vi "test - Empty String Check.vi"(8 "error in (no error)":errorcluster, 11 "TestCase in":refnum<class "testcase-Supported-Datatype.lvclass">) -> (0 "error out":errorcluster, 3 "TestCase out":refnum<class "testcase-Supported-Datatype.lvclass">)   [LabVIEW 2017, in "testcase-Supported-Datatype.lvclass"]
uses:
  testcase-Supported-Datatype.lvclass
  <vilib>/addons/_JKI Toolkits/VI Tester/TestCase.llb/TestCase.lvclass
  addons/API-String-Arugments-Support/API String Arguments Support.lvlib
  C:/Program Files (x86)/National Instruments/LabVIEW 2017/vi.lib/addons/_JKI Toolkits/VI Tester/TestCase.llb/TestCase.lvclass
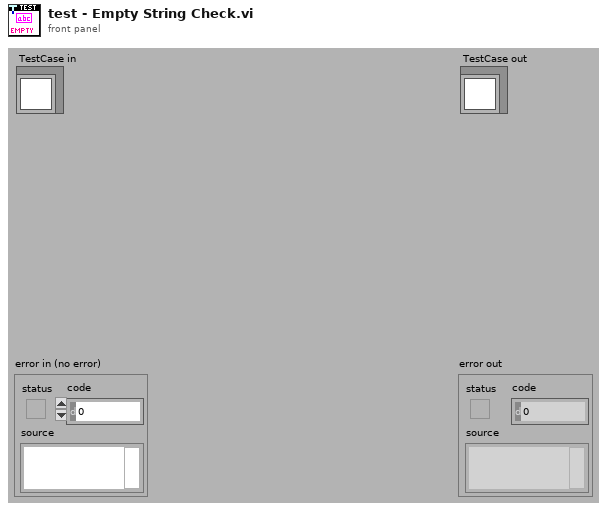
[diagram p1: front panel]
types:
  T1 = cluster{"Name":string, "Child":cluster{"Name":string}, "Bool":bool}[]
  T2 = cluster{"Name":string, "Child":cluster{"Name":string}, "Bool":bool}
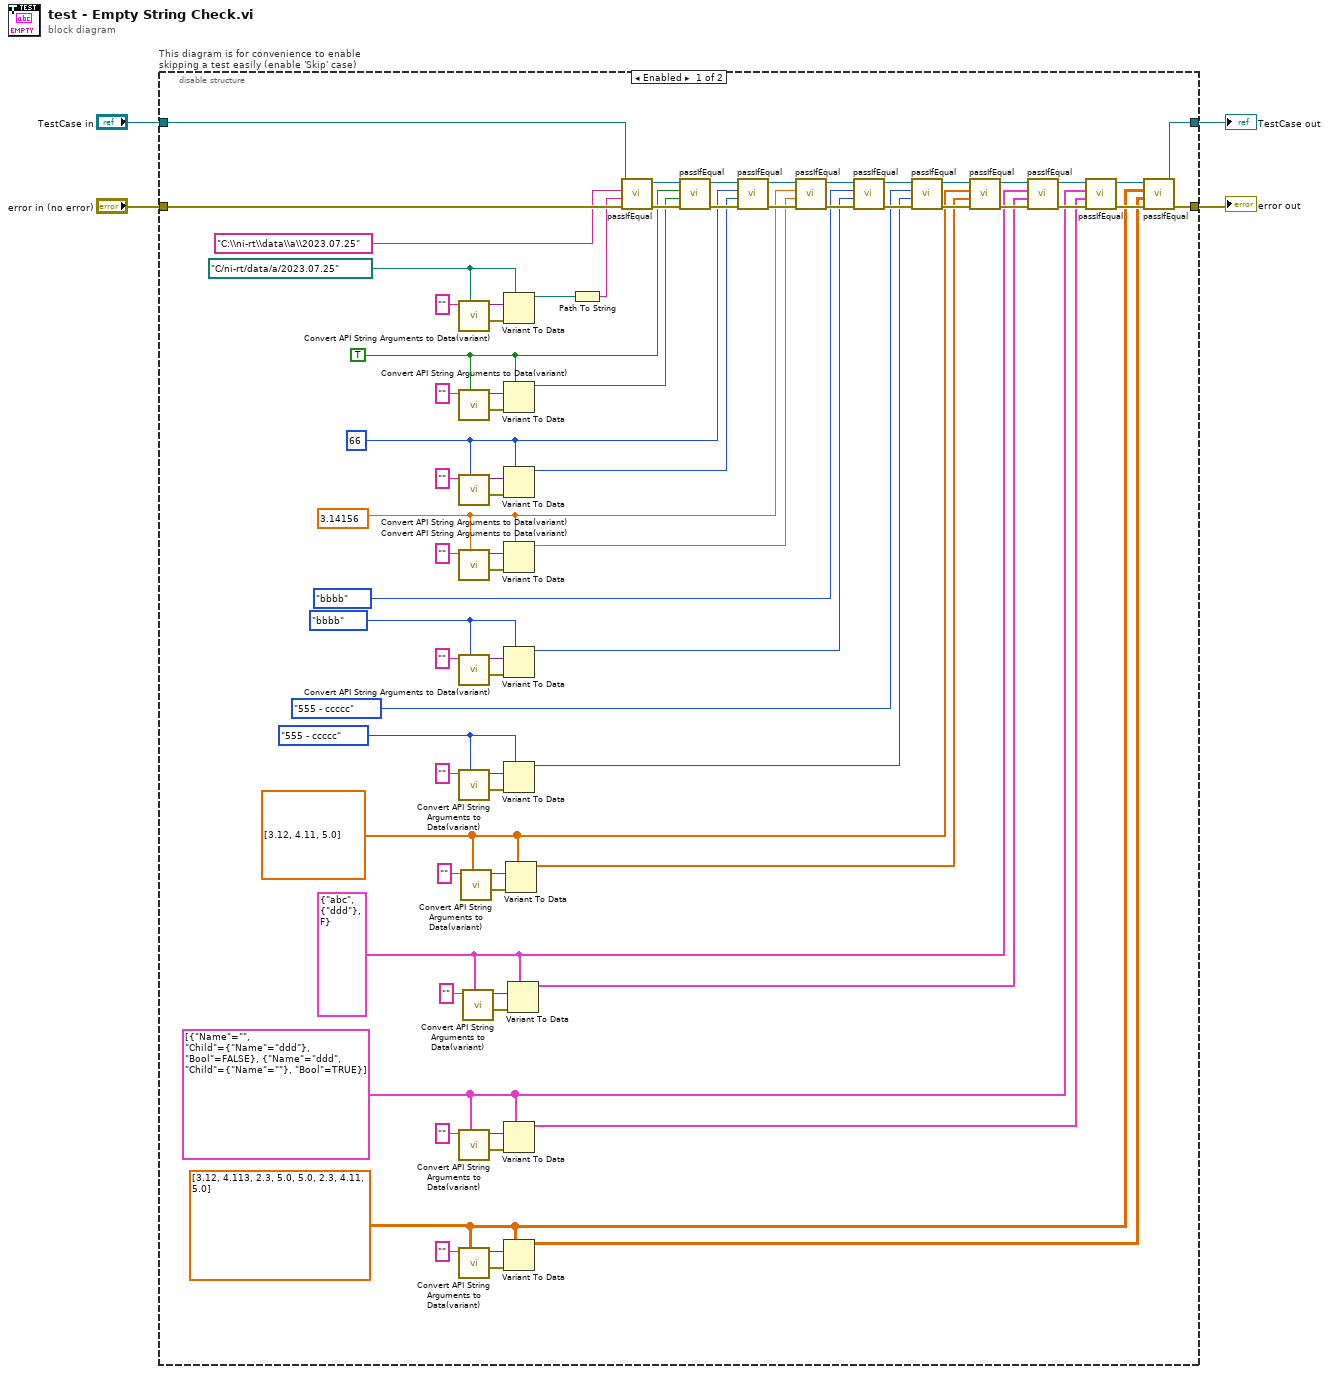
[diagram p0: block diagram]
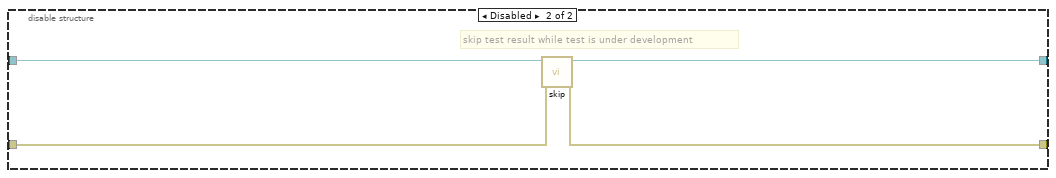
[diagram p2: hidden frame]
diagram:
  n1 = disable-structure "This diagram is for convenience to enable skipping a test easily (enable 'Skip' case)" shown="Enabled" {
    disable-tunnel: "TestCase in" -> [w80 w84]
    disable-tunnel: [w5 w82] -> w1
    disable-tunnel: [w6 w83] -> w3
    disable-tunnel: "error in (no error)" -> [w79 w81]
    frame Enabled {
      w8 = dbl[][] [[3.12, 4.113, 2.3, 5.0, 5.0, 2.3, 4.11, 5.0]] ("Data 11")
      w15 = T1 [{"Name"="", "Child"={"Name"="ddd"}, "Bool"=FALSE}, {"Name"="ddd", "Child"={"Name"=""}, "Bool"=TRUE}] ("Data 10")
      w22 = T2 {"Name"="abc", "Child"={"Name"="ddd"}, "Bool"=FALSE} ("Data 8")
      w29 = dbl[] [3.12, 4.11, 5.0] ("Data 4")
      w39 = enum16{"1 - aaaa", "2 - bbbb", "555 - ccccc"}."555 - ccccc" ("Data 6")
      w47 = enum16{"aaaa", "bbbb", "ccccc"}."bbbb" ("Data 5")
      w52 = 3.14156
      w59 = 66
      w66 = TRUE
      w75 = path "C:/ni-rt/data/a/2023.07.25" ("Data 9")
      n2 = call "Convert API String Arguments to Data(variant).vi"("Type"=w75, "String"="") -> ("error"=w78:errorcluster, "Data"=w77:variant)  [unwired: 8 in]
      n3 = call "Convert API String Arguments to Data(variant).vi"("Type"=w66, "String"="") -> ("error"=w71:errorcluster, "Data"=w70:variant)  [unwired: 8 in]
      n4 = call "Convert API String Arguments to Data(variant).vi"("Type"=w59, "String"="") -> ("error"=w62:errorcluster, "Data"=w63:variant)  [unwired: 8 in]
      n5 = call "Convert API String Arguments to Data(variant).vi"("Type"=w52, "String"="") -> ("error"=w57:errorcluster, "Data"=w56:variant)  [unwired: 8 in]
      n6 = call "Convert API String Arguments to Data(variant).vi"("Type"=w47, "String"="") -> ("error"=w50:errorcluster, "Data"=w49:variant)  [unwired: 8 in]
      n7 = call "Convert API String Arguments to Data(variant).vi"("Type"=w39, "String"="") -> ("error"=w40:errorcluster, "Data"=w41:variant)  [unwired: 8 in]
      n8 = call "Convert API String Arguments to Data(variant).vi"("Type"=w15, "String"="") -> ("error"=w20:errorcluster, "Data"=w19:variant)  [unwired: 8 in]
      n9 = call "Convert API String Arguments to Data(variant).vi"("Type"=w8, "String"="") -> ("error"=w11:errorcluster, "Data"=w12:variant)  [unwired: 8 in]
      n10 = call "Convert API String Arguments to Data(variant).vi"("Type"=w29, "String"="") -> ("error"=w34:errorcluster, "Data"=w33:variant)  [unwired: 8 in]
      n11 = call "Convert API String Arguments to Data(variant).vi"("Type"=w22, "String"="") -> ("error"=w25:errorcluster, "Data"=w26:variant)  [unwired: 8 in]
      n12 = Variant To Data(error in=w78, type=w75, Variant=w77) -> (data=w74:path)  [unwired: 1 out]
      n13 = Variant To Data(error in=w71, type=w66, Variant=w70) -> (data=w65:bool)  [unwired: 1 out]
      n14 = Variant To Data(error in=w62, type=w59, Variant=w63) -> (data=w58:i32)  [unwired: 1 out]
      n15 = Variant To Data(error in=w57, type=w52, Variant=w56) -> (data=w51:dbl)  [unwired: 1 out]
      n16 = Variant To Data(error in=w50, type=w47, Variant=w49) -> (data=w43:enum16{"aaaa", "bbbb", "ccccc"})  [unwired: 1 out]
      n17 = Variant To Data(error in=w40, type=w39, Variant=w41) -> (data=w35:enum16{"1 - aaaa", "2 - bbbb", "555 - ccccc"})  [unwired: 1 out]
      n18 = Variant To Data(error in=w20, type=w15, Variant=w19) -> (data=w14:T1)  [unwired: 1 out]
      n19 = Variant To Data(error in=w11, type=w8, Variant=w12) -> (data=w7:dbl[][])  [unwired: 1 out]
      n20 = Variant To Data(error in=w34, type=w29, Variant=w33) -> (data=w28:dbl[])  [unwired: 1 out]
      n21 = Variant To Data(error in=w25, type=w22, Variant=w26) -> (data=w21:T2)  [unwired: 1 out]
      n22 = Path To String(path=w74) -> (string=w72:string)
      n23 = call-dynamic "passIfEqual.vi"("error in (no error)"=w79, "y"=w72, "x"="C:\\ni-rt\\data\\a\\2023.07.25" ("String 10"), "TestCase in"=w80) -> ("error out"=w68:errorcluster, "TestCase out"=w67:refnum<class "testcase-Supported-Datatype.lvclass">)  [unwired: 6 in]
      n24 = call-dynamic "passIfEqual.vi"("error in (no error)"=w68, "y"=w65, "x"=w66, "TestCase in"=w67) -> ("error out"=w61:errorcluster, "TestCase out"=w60:refnum<class "testcase-Supported-Datatype.lvclass">)  [unwired: 6 in]
      n25 = call-dynamic "passIfEqual.vi"("error in (no error)"=w61, "y"=w58, "x"=w59, "TestCase in"=w60) -> ("error out"=w53:errorcluster, "TestCase out"=w54:refnum<class "testcase-Supported-Datatype.lvclass">)  [unwired: 6 in]
      n26 = call-dynamic "passIfEqual.vi"("error in (no error)"=w53, "y"=w51, "x"=w52, "TestCase in"=w54) -> ("error out"=w46:errorcluster, "TestCase out"=w45:refnum<class "testcase-Supported-Datatype.lvclass">)  [unwired: 6 in]
      n27 = call-dynamic "passIfEqual.vi"("error in (no error)"=w46, "y"=w43, "x"=enum16{"aaaa", "bbbb", "ccccc"}."bbbb" ("Data 5"), "TestCase in"=w45) -> ("error out"=w38:errorcluster, "TestCase out"=w37:refnum<class "testcase-Supported-Datatype.lvclass">)  [unwired: 6 in]
      n28 = call-dynamic "passIfEqual.vi"("error in (no error)"=w38, "y"=w35, "x"=enum16{"1 - aaaa", "2 - bbbb", "555 - ccccc"}."555 - ccccc" ("Data 6"), "TestCase in"=w37) -> ("error out"=w30:errorcluster, "TestCase out"=w31:refnum<class "testcase-Supported-Datatype.lvclass">)  [unwired: 6 in]
      n29 = call-dynamic "passIfEqual.vi"("error in (no error)"=w30, "y"=w28, "x"=w29, "TestCase in"=w31) -> ("error out"=w23:errorcluster, "TestCase out"=w24:refnum<class "testcase-Supported-Datatype.lvclass">)  [unwired: 6 in]
      n30 = call-dynamic "passIfEqual.vi"("error in (no error)"=w23, "y"=w21, "x"=w22, "TestCase in"=w24) -> ("error out"=w16:errorcluster, "TestCase out"=w17:refnum<class "testcase-Supported-Datatype.lvclass">)  [unwired: 6 in]
      n31 = call-dynamic "passIfEqual.vi"("error in (no error)"=w16, "y"=w14, "x"=w15, "TestCase in"=w17) -> ("error out"=w9:errorcluster, "TestCase out"=w10:refnum<class "testcase-Supported-Datatype.lvclass">)  [unwired: 6 in]
      n32 = call-dynamic "passIfEqual.vi"("error in (no error)"=w9, "y"=w7, "x"=w8, "TestCase in"=w10) -> ("error out"=w6:errorcluster, "TestCase out"=w5:refnum<class "testcase-Supported-Datatype.lvclass">)  [unwired: 6 in]
    }
    frame Disabled {
      # "skip test result while test is under development"
      n33 = call <vilib>:"skip.vi"("error in (no error)"=w81, "TestCase in"=w84) -> ("error out"=w83:errorcluster, "TestCase out"=w82:refnum<class "testcase-Supported-Datatype.lvclass">)  [unwired: 8 in]
    }
  }
  "error out" <- w3
  "TestCase out" <- w1
